vi "BDF-Open For Playback.vi"(0 "Header":T1, 11 "error in (no error)":errorcluster) -> (4 "Header thru":T1, 6 "refnum out":refnum<file>, 15 "error out":errorcluster)   [LabVIEW 2020]
uses:
  BDF-Header.ctl
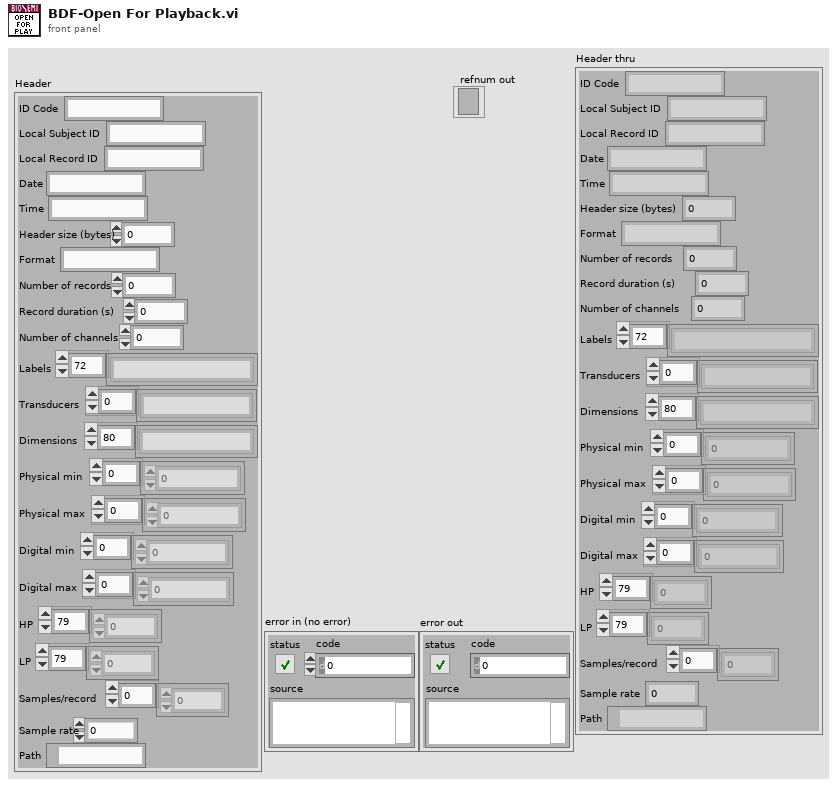
[diagram p1: front panel]
types:
  T1 = typedef "BDF-Header.ctl" = cluster{"ID Code":string, "Local Subject ID":string, "Local Record ID":string, "Date":string, "Time":string, "Header size (bytes)":i32, "Format":string, "Number of records":i32, "Record duration (s)":dbl, "Number of channels":i32, "Labels":string[], "Transducers":string[], "Dimensions":string[], "Physical min":dbl[], "Physical max":dbl[], "Digital min":i32[], "Digital max":i32[], "HP":dbl[], "LP":dbl[], "Samples/record":i32[], "Sample rate":dbl, "Path":path}
  T2 = enum16{"open", "replace", "create", "open or create", "replace or create", "replace or create with confirmation"}
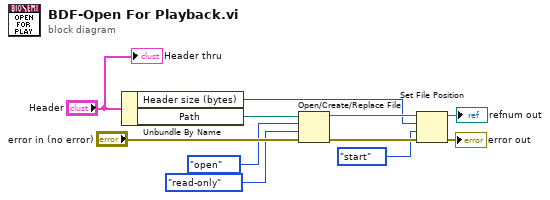
[diagram p0: block diagram]
diagram:
  n1 = Unbundle By Name("Header") -> ("Header size (bytes)"=w5:i32, "Path"=w1:path)
  n2 = Open/Create/Replace File(file path (use dialog)=w1, error in="error in (no error)", operation (0:open)=T2."open", access (0:read/write)=enum16{"read/write", "read-only", "write-only"}."read-only") -> (refnum out=w7:refnum<file>, error out=w8:errorcluster)  [unwired: 2 in, 1 out]
  n3 = Set File Position(offset (in bytes) (0)=w5, refnum=w7, from (0:start)=enum16{"start", "end", "current"}."start", error in=w8) -> (refnum out=→"refnum out":refnum<file>, error out=→"error out":errorcluster)
  "Header thru" <- "Header"
